vi "Helper-SubPanel.vi"() -> ()   [LabVIEW 2016]
panel:
  in  "Load SP1":bool
  in  "Remove":bool
  out "error out":errorcluster
  in  "stop":bool
  in  "Load SP2":bool
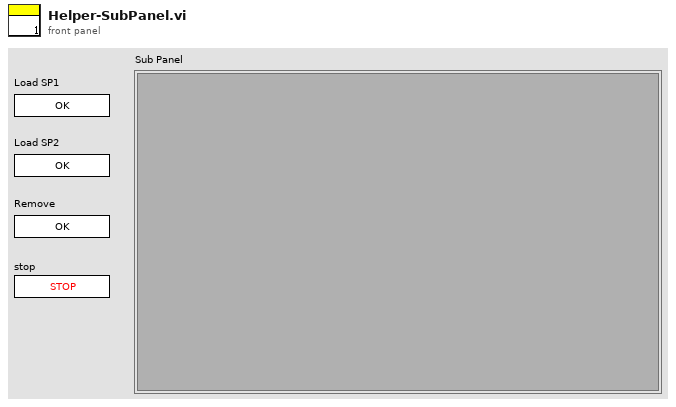
[diagram p1: front panel]
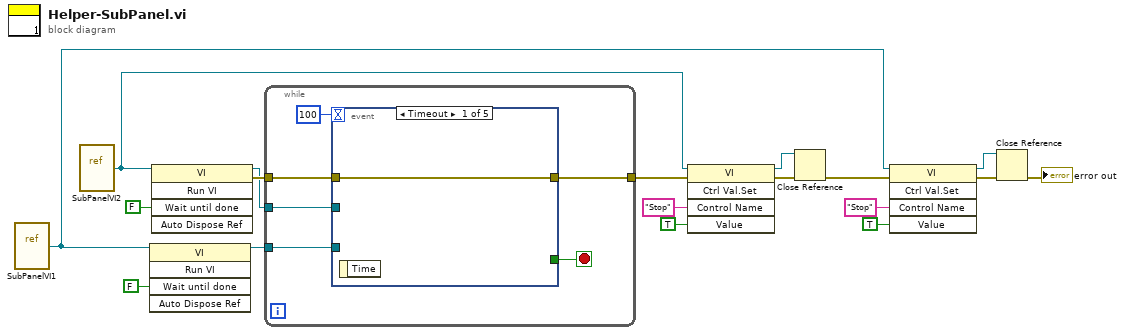
[diagram p0: block diagram]
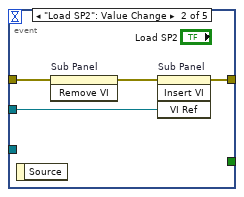
[diagram p2: hidden frame]
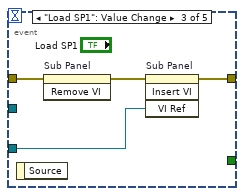
[diagram p3: hidden frame]
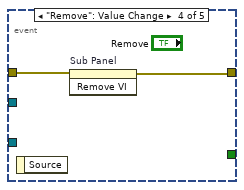
[diagram p4: hidden frame]
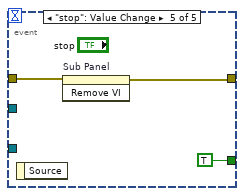
[diagram p5: hidden frame]
diagram:
  n1 = vi-ref "SubPanelVI1.vi"() -> (w2:refnum<vi>)
  n2 = vi-ref "SubPanelVI2.vi"() -> (w10:refnum<vi>)
  n3 = invoke class="VI" method="Run VI"(reference=w2, "Wait until done"=FALSE ("Wait Until Done")) -> (reference out=w14:refnum<vi>)  [unwired: 3 in, 4 out]
  n4 = invoke class="VI" method="Run VI"(reference=w10, "Wait until done"=FALSE ("Wait Until Done")) -> (reference out=w17:refnum<vi>, error out=w18:errorcluster)  [unwired: 3 in, 3 out]
  n5 = while {
    tunnel: w18 -> [w23]
    tunnel: [w22] -> w11
    tunnel: w17 -> [w21]
    tunnel: w14 -> [w20]
    stop <- w19 stop-if-true
    n6 = event shown="[0] Timeout" {
      selector: _ -> [_ _ _ _ _]
      dyn-events: _ -> [_ _ _ _ _]
      timeout: 100 -> [_ _ _ _ _]
      tunnel: w23 -> [w25 w27 w31 w35 w38]
      tunnel: [w25 w28 w33 w34 w37] -> w22
      tunnel: w21 -> [_ w29 _ _ _]
      tunnel: w20 -> [_ _ w32 _ _]
      tunnel: [_ _ _ _ TRUE ("stop")] -> w19
      event Timeout {
        n7 = event-data() -> ()  [unwired: 1 in, 1 out]
      }
      event "Load SP2": Value Change {
        n8 = event-data() -> ()  [unwired: 1 in, 1 out]
        n9 = invoke on="Sub Panel" class="SubPnl" method="Remove VI"(error in=w27) -> (error out=w26:errorcluster)  [unwired: 2 in, 2 out]
        n10 = invoke on="Sub Panel" class="SubPnl" method="Insert VI"(error in=w26, "VI Ref"=w29) -> (error out=w28:errorcluster)  [unwired: 2 in, 3 out]
      }
      event "Load SP1": Value Change {
        n11 = event-data() -> ()  [unwired: 1 in, 1 out]
        n12 = invoke on="Sub Panel" class="SubPnl" method="Remove VI"(error in=w31) -> (error out=w30:errorcluster)  [unwired: 2 in, 2 out]
        n13 = invoke on="Sub Panel" class="SubPnl" method="Insert VI"(error in=w30, "VI Ref"=w32) -> (error out=w33:errorcluster)  [unwired: 2 in, 3 out]
      }
      event "Remove": Value Change {
        n14 = event-data() -> ()  [unwired: 1 in, 1 out]
        n15 = invoke on="Sub Panel" class="SubPnl" method="Remove VI"(error in=w35) -> (error out=w34:errorcluster)  [unwired: 2 in, 2 out]
      }
      event "stop": Value Change {
        n16 = event-data() -> ()  [unwired: 1 in, 1 out]
        n17 = invoke on="Sub Panel" class="SubPnl" method="Remove VI"(error in=w38) -> (error out=w37:errorcluster)  [unwired: 2 in, 2 out]
      }
    }
  }
  n18 = invoke class="VI" method="Ctrl Val.Set"(reference=w10, error in=w11, "Control Name"="Stop", "Value"=TRUE) -> (reference out=w8:refnum<vi>, error out=w9:errorcluster)  [unwired: 1 in, 3 out]
  n19 = Close Reference(reference=w8, error in (no error)=w9) -> (error out=w3:errorcluster)
  n20 = invoke class="VI" method="Ctrl Val.Set"(reference=w2, error in=w3, "Control Name"="Stop", "Value"=TRUE) -> (reference out=w7:refnum<vi>, error out=w6:errorcluster)  [unwired: 1 in, 3 out]
  n21 = Close Reference(reference=w7, error in (no error)=w6) -> (error out=→"error out":errorcluster)
